vi "Memory.Array.New.vi"(7 "allocation limit (2^31: 2GiB)":i64=2147483647 format="%08x bytes", 8 "error in (no error)":errorcluster, 9 "number of elements":u64, 10 "size of element":i64 format="%d bytes") -> (0 "error out":errorcluster, 3 "Array out":refnum<class "Memory.Array.lvclass">)   [LabVIEW 2016, in "LabVIEW Memory Manager.lvlib" / "Memory.Array.lvclass"]
uses:
  Memory.Array.lvclass
  Pointer/Memory.Pointer.lvclass/Memory.Pointer.ctl
  Memory.Array.lvclass/Memory.Array.ctl
  Memory.Array.Set Pointer.vi
  Memory.Array.Set Element Size.vi
  Memory.Array.Set Number of Elements.vi
  Pointer/Methods/Memory.Pointer.New.vi
  Pointer/Methods/Memory.Pointer.Allocate.vi
  Pointer/Methods/Accessors/Memory.Pointer.Set Address.vi
  Pointer/Methods/Accessors/Memory.Pointer.Set Size.vi
  Pointer/Methods/Memory.Pointer.Parameter Check.Size.vi
  Pointer/Memory.Pointer.lvclass
panel:
  out "allocated size":i64 format="%d bytes"
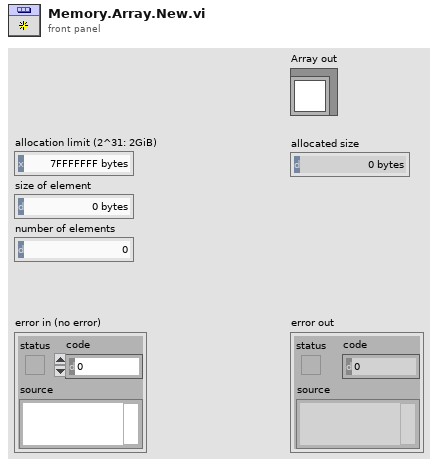
[diagram p1: front panel]
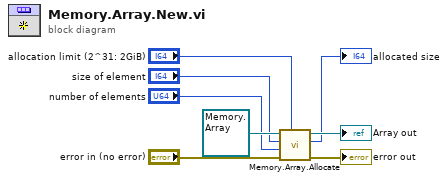
[diagram p0: block diagram]
diagram:
  n1 = call "Memory.Array.Allocate.vi"("allocation limit (2^31: 2GiB)"="allocation limit (2^31: 2GiB)", "error in (no error)"="error in (no error)", "number of elements"="number of elements", "size of element"="size of element", "Array in"=refnum<class "Memory.Array.lvclass"> refnum) -> ("error out"=→"error out":errorcluster, "allocated size"=→"allocated size":i64, "Array out"=→"Array out":refnum<class "Memory.Array.lvclass">)  [unwired: 4 in]
